vi "_PC_D999_get_param.vi"(7 "stop cmd":refnum<data-value>, 8 "error in (no error)":errorcluster, 11 "D999_exist SV":refnum<k21>) -> (0 "error out":errorcluster, 3 "D999_Param":T1={"Enable"=FALSE, "AI"=[{"Label"="", "MultiValue"=1.0, "AddValue"=0.0}, {"Label"="", "MultiValue"=1.0, "AddValue"=0.0}, {"Label"="", "MultiValue"=1.0, "AddValue"=0.0}, {"Label"="", "MultiValue"=1.0, "AddValue"=0.0}, {"Label"="", "MultiValue"=1.0, "AddValue"=0.0}, {"Label"="", "MultiValue"=1.0, "AddValue"=0.0}, {"Label"="", "MultiValue"=1.0, "AddValue"=0.0}, {"Label"="", "MultiValue"=1.0, "AddValue"=0.0}, {"Label"="", "MultiValue"=1.0, "AddValue"=0.0}, {"Label"="", "MultiValue"=1.0, "AddValue"=0.0}, {"Label"="", "MultiValue"=1.0, "AddValue"=0.0}, {"Label"="", "MultiValue"=1.0, "AddValue"=0.0}], "AO"=[], "Switch"=[]})   [LabVIEW 2018]
uses:
  RT/PublicSubVI/Ctl/_ctl_RT_D999_Param.ctl
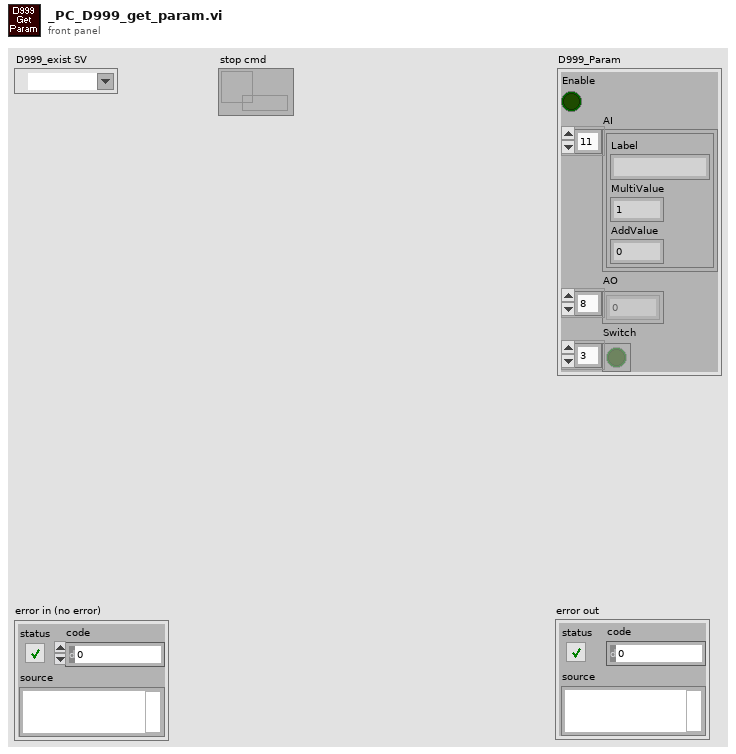
[diagram p1: front panel]
types:
  T1 = typedef "_ctl_RT_D999_Param.ctl" = cluster{"Enable":bool, "AI":cluster{"Label":string, "MultiValue":dbl, "AddValue":dbl}[], "AO":i16[], "Switch":bool[]}
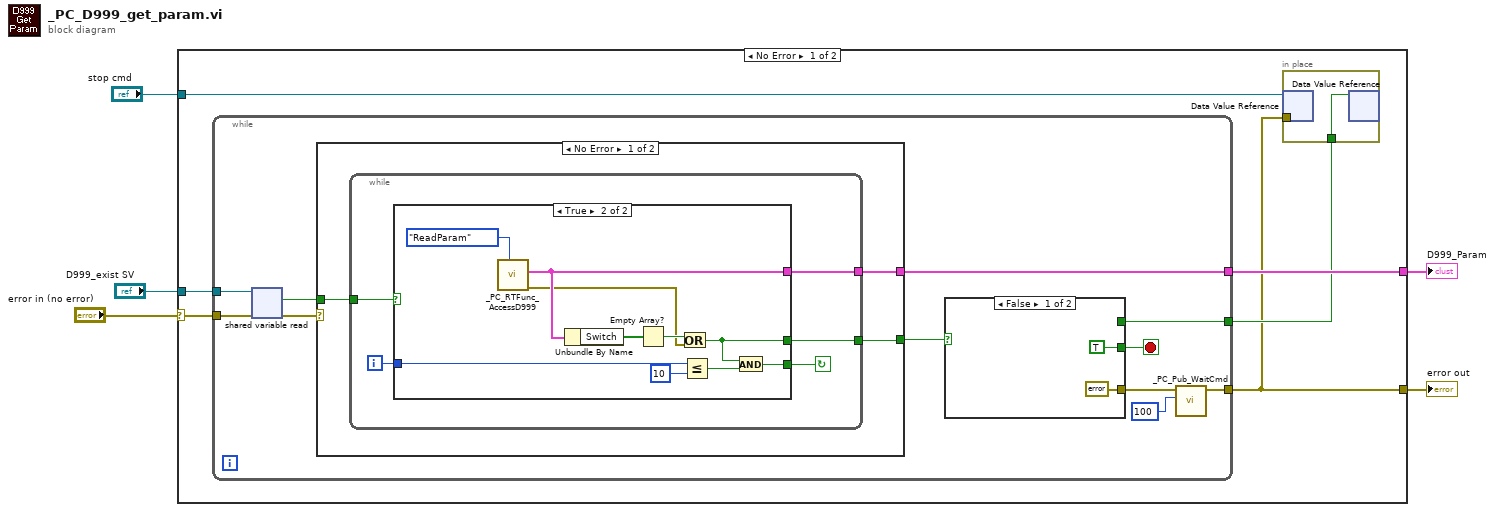
[diagram p0: block diagram]
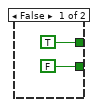
[diagram p2: hidden frame]
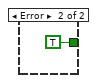
[diagram p3: hidden frame]
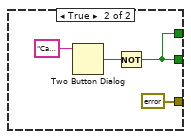
[diagram p4: hidden frame]
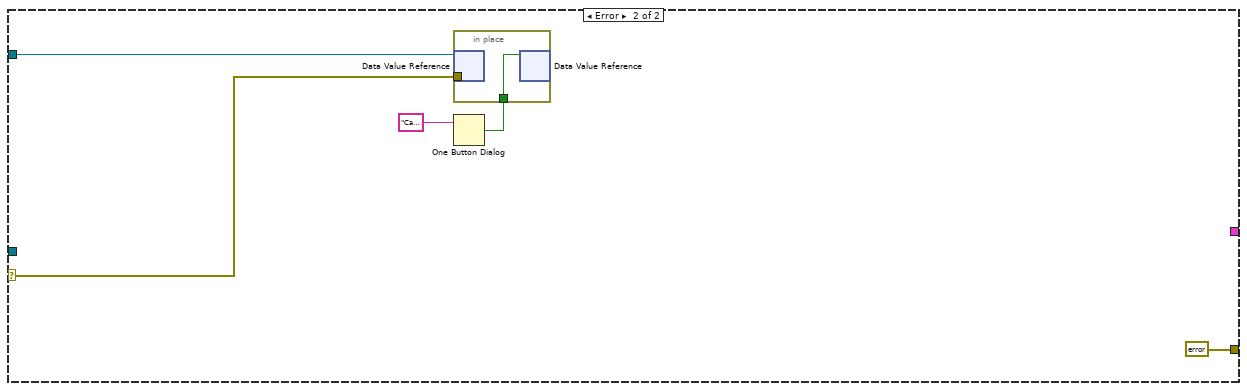
[diagram p5: hidden frame]
diagram:
  n1 = case shown="No Error" "error in (no error)" {
    selector: "error in (no error)" -> [w9 w54]
    tunnel: [w6 errorcluster {"status"=TRUE, "code"=0, "source"=""} ("error in")] -> w5
    tunnel: [w11 _] -> w4
    tunnel: "D999_exist SV" -> [w10 _]
    tunnel: "stop cmd" -> [w8 w55]
    frame No Error {
      n2 = while {
        tunnel: [w18] -> w6
        tunnel: [w21] -> w11
        tunnel: w10 -> [w17]
        tunnel: w9 -> [w16]
        tunnel: [w13] -> w7
        stop <- w23 stop-if-true
        n3 = shared-variable-read(w17, w16) -> (w15:errorcluster, w14:bool)  [unwired: 1 out]
        n4 = case shown="No Error" w15 {
          tunnel: w14 -> [w26 _]
          tunnel: [w25 _] -> w21
          tunnel: [w24 TRUE] -> w22
          frame No Error {
            n5 = while {
              tunnel: w26 -> [w31]
              tunnel: [w30] -> w24
              tunnel: [w27] -> w25
              i -> [w28]
              stop <- w29 continue-if-true
              n6 = case shown="True" w31 {
                tunnel: [TRUE w34] -> w30
                tunnel: [FALSE w35] -> w29
                tunnel: w28 -> [_ w43]
                tunnel: [_ w38] -> w27
                frame False {
                }
                frame True {
                  n7 = call "_PC_RTFunc_AccessD999.vi"("Function"=enum16{"WriteCmd", "ReadParam", "ReadResponse"}."ReadParam") -> ("error out"=w37:errorcluster, "D999_Param"=w38:T1)  [unwired: 9 in]
                  n8 = Unbundle By Name(w38) -> ("Switch"=w40:bool[])
                  n9 = Empty Array?(array=w40) -> (empty?=w39:bool)
                  n10 = Or(x=w39, y=w37) -> (x .or. y?=w34:bool)
                  n11 = Less Or Equal?(x=w43, y=10) -> (x <= y?=w36:bool)
                  n12 = And(x=w34, y=w36) -> (x .and. y?=w35:bool)
                }
              }
            }
          }
          frame Error {
          }
        }
        n13 = case shown="False" w22 {
          tunnel: [TRUE w47] -> w23
          tunnel: [errorcluster {"status"=FALSE, "code"=0, "source"=""} ("error in") errorcluster {"status"=TRUE, "code"=0, "source"=""} ("error in")] -> w19
          tunnel: [_ w47] -> w13
          frame False {
          }
          frame True {
            n14 = Two Button Dialog(message="Can't Find D999.\nReCheck?") -> (T button?=w50:bool)  [unwired: 2 in]
            n15 = Not(x=w50) -> (.not. x?=w47:bool)
          }
        }
        n16 = call "_PC_Pub_WaitCmd.vi"("milliseconds to wait"=u32 100, "error in (no error)"=w19) -> ("error out"=w18:errorcluster)  [unwired: 9 in]
      }
      n17 = in-place {
        in-place-border: w7 -> [w12]
        in-place-border: w6 -> [_]
        n18 = in-place-dvr #1(w8) -> ()  [unwired: 2 out]
        n19 = in-place-dvr #1(w12) -> ()  [unwired: 2 out]
      }
    }
    frame Error {
      n20 = One Button Dialog(message="Can't Find D999.\nReCheck?") -> (true=w52:bool)  [unwired: 1 in]
      n21 = in-place {
        in-place-border: w54 -> [_]
        in-place-border: w52 -> [w56]
        n22 = in-place-dvr #2(w55) -> ()  [unwired: 2 out]
        n23 = in-place-dvr #2(w56) -> ()  [unwired: 2 out]
      }
    }
  }
  "error out" <- w5
  "D999_Param" <- w4
